vi "Autonomous Independent.vi"   [LabVIEW 2014]
doc: "This VI is called when autonomous begins, and will automatically be terminated when autonomous ends. You can carry out timed or sensor driven robot movement independently without needing to return to the caller."
uses:
  TypeDefs/SRE Enum.ctl
  Robot Global Data.vi
panel:
  # "Be sure to right-click and choose Data Operations>>Make Current Value default if you want to save the array values with the VI"
types:
  T1 = typedef "SRE Enum.ctl" = enum16{"Start", "Run", "End"}
  T2 = enum16{"Center to 0", "Center to -45", "Center to 45"}
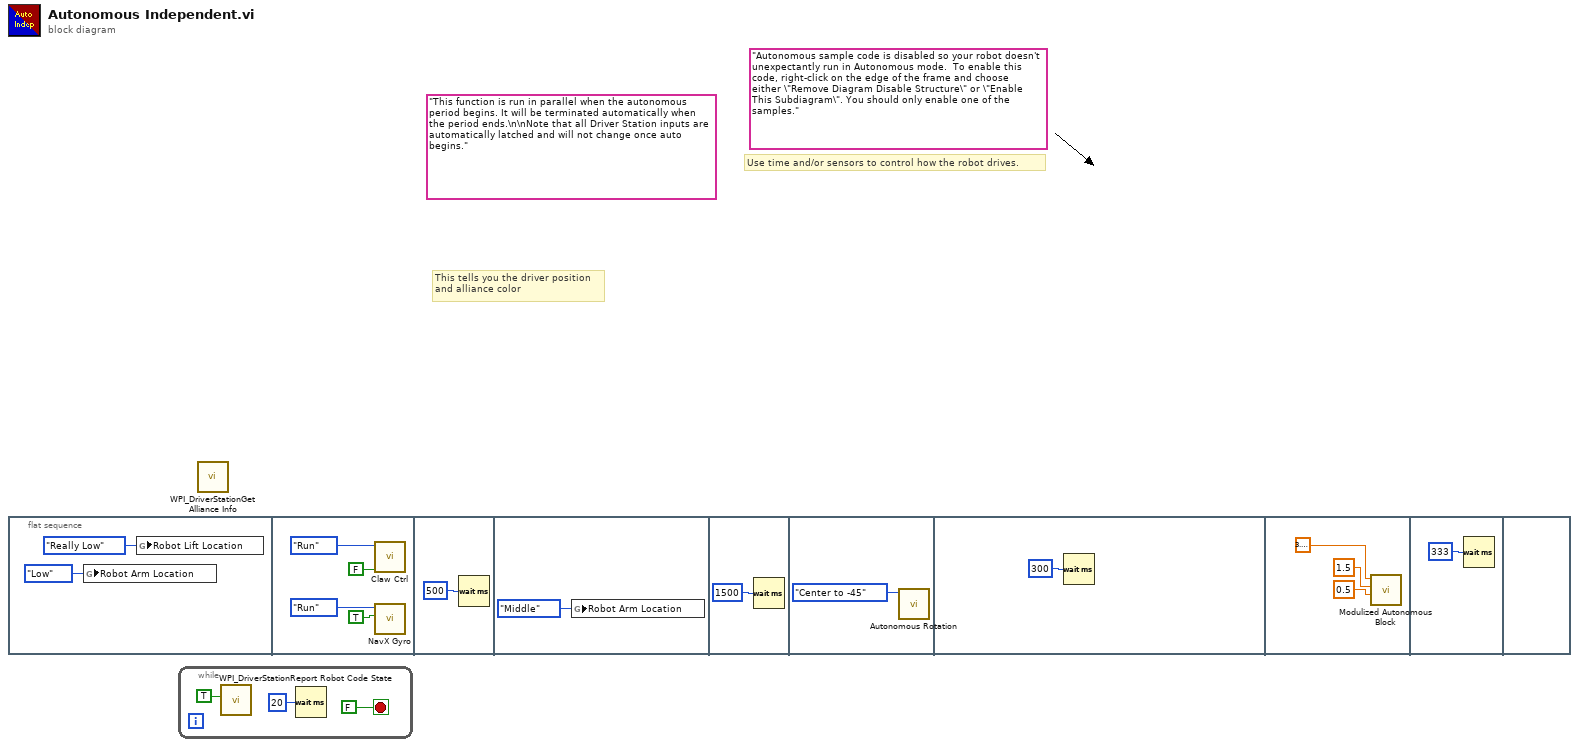
[diagram p0: block diagram]
diagram:
  (unwired) "Autonomous sample code is disabled so your robot doesn't unexpectantly run in Autonomous mode.  To enable this code, right-click on the edge of the frame and choose either \"Remove Diagram Disable Structure\" or \"Enable This Subdiagram\". You should only enable one of the samples."
  (unwired) "This function is run in parallel when the autonomous period begins. It will be terminated automatically when the period ends.\n\nNote that all Driver Station inputs are automatically latched and will not change once auto begins."
  # "Use time and/or sensors to control how the robot drives."
  # "This tells you the driver position\nand alliance color"
  n1 = flat-sequence {
    frame #0 {
      n2 = global write "Robot Global Data.vi" "Robot Arm Location"(enum16{"High", "Middle", "Low"}."Low" ("Robot Arm Location")) -> ()
      n3 = global write "Robot Global Data.vi" "Robot Lift Location"(enum16{"High", "Middle", "Low", "Really Low"}."Really Low" ("Robot Lift Location")) -> ()
    }
    frame #1 {
      n4 = call "Claw Ctrl.vi"("Open/Close"=FALSE, "Enum"=SRE_Enum."Run") -> ()  [unwired: 10 in]
      n5 = call "NavX Gyro.vi"("Reset"=TRUE, "Enum"=SRE_Enum."Run") -> ()  [unwired: 8 in, 2 out]
    }
    frame #2 {
      n6 = Wait (ms)(milliseconds to wait=u32 500) -> ()  [unwired: 1 out]
    }
    frame #3 {
      n7 = global write "Robot Global Data.vi" "Robot Arm Location"(enum16{"High", "Middle", "Low"}."Middle" ("Robot Arm Location")) -> ()
    }
    frame #4 {
      n8 = Wait (ms)(milliseconds to wait=u32 1500) -> ()  [unwired: 1 out]
    }
    frame #5 {
      n9 = call "Autonomous Rotation.vi"("center Options"=T2."Center to -45") -> ()  [unwired: 11 in]
    }
    frame #6 {
      n10 = Wait (ms)(milliseconds to wait=u32 300) -> ()  [unwired: 1 out]
    }
    frame #7 {
      n11 = call "Modulized Autonomous Block.vi"("Power"=0.5, "run time in seconds"=1.5 ("Direction"), "Direction"=3.141592653589793) -> ()  [unwired: 8 in, 1 out]
    }
    frame #8 {
      n12 = Wait (ms)(milliseconds to wait=u32 333) -> ()  [unwired: 1 out]
    }
    frame #9 {
    }
  }
  n13 = while {
    stop <- FALSE stop-if-true
    n14 = call <vilib>:"WPI_DriverStationReport Robot Code State.vi"("Autonomous"=TRUE) -> ()  [unwired: 10 in, 1 out]
    n15 = Wait (ms)(milliseconds to wait=u32 20) -> ()  [unwired: 1 out]
  }
  n16 = call <vilib>:"WPI_DriverStationGet Alliance Info.vi"() -> ()  [unwired: 12 out]
